vi "Traverse Cluster.vi"(10 "Nest Chain":string[](array[string]), 11 "Data Type":variant) -> (3 "Array":T1[](array[typedef]))   [LabVIEW 2023]
doc: "Reentrant VI recursively returns references of controls in a cluster and compiles data needed for display in tree, such as the nesting heirarchy of nested clusters."
uses:
  Cluster Element Description.ctl
  <vilib>/Utility/Data Type/NI_Data Type.lvlib
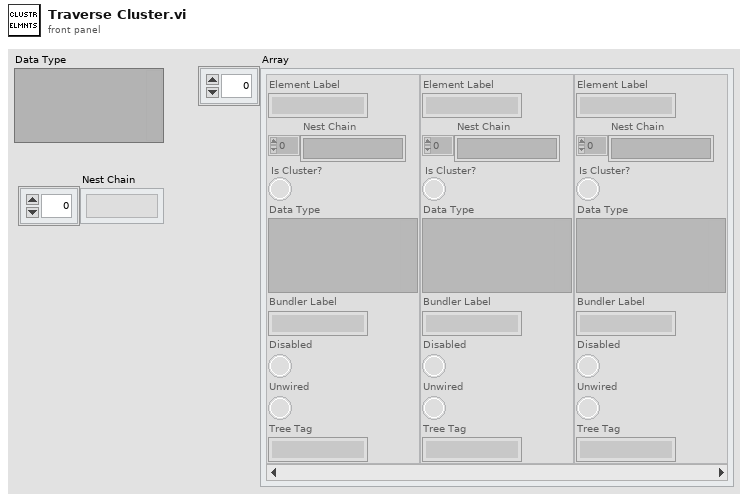
[diagram p1: front panel]
types:
  T1 = typedef "Cluster Element Description.ctl" = cluster{"Element Label":string, "Nest Chain":string[], "Is Cluster?":bool, "Data Type":variant, "Bundler Label":string, "Disabled":bool, "Unwired":bool, "Tree Tag":string}
  T2 = enum8{"Invalid Type", "Void", "I8", "I16", "I32", "I64", "U8", "U16", "U32", "U64", "Single Float", "Double Float", "Extended Float", "Single Complex", "Double Complex", "Extended Complex", "Enum U8", "Enum U16", "Enum U32", "Enum U64", "Single Float With Unit", "Double Float With Unit", "Extended Float With Unit", "Single Complex with Unit", "Double Complex with Unit", "Extended Complex with Unit", "Boolean", "String", "Path", "Picture", "Tag", "Array", "Cluster", "Variant", "LV Variant", "Waveform", "Timestamp", "Digital Waveform", "Digital Data", "ExpressData", "Refnum", "External Data", "VI", "Poly VI", "LabVIEW Class Instance", "Fixed Point"}
  T3 = typedef "NI_Data Type.lvlib/Data Type.ctl" = enum8{"Invalid Type", "Void", "I8", "I16", "I32", "I64", "U8", "U16", "U32", "U64", "Single Float", "Double Float", "Extended Float", "Single Complex", "Double Complex", "Extended Complex", "Enum U8", "Enum U16", "Enum U32", "Enum U64", "Single Float With Unit", "Double Float With Unit", "Extended Float With Unit", "Single Complex with Unit", "Double Complex with Unit", "Extended Complex with Unit", "Boolean", "String", "Path", "Picture", "Tag", "Array", "Cluster", "Variant", "LV Variant", "Waveform", "Timestamp", "Digital Waveform", "Digital Data", "ExpressData", "Refnum", "External Data", "VI", "Poly VI", "LabVIEW Class Instance", "Fixed Point", "Set Collection", "Map Collection"}
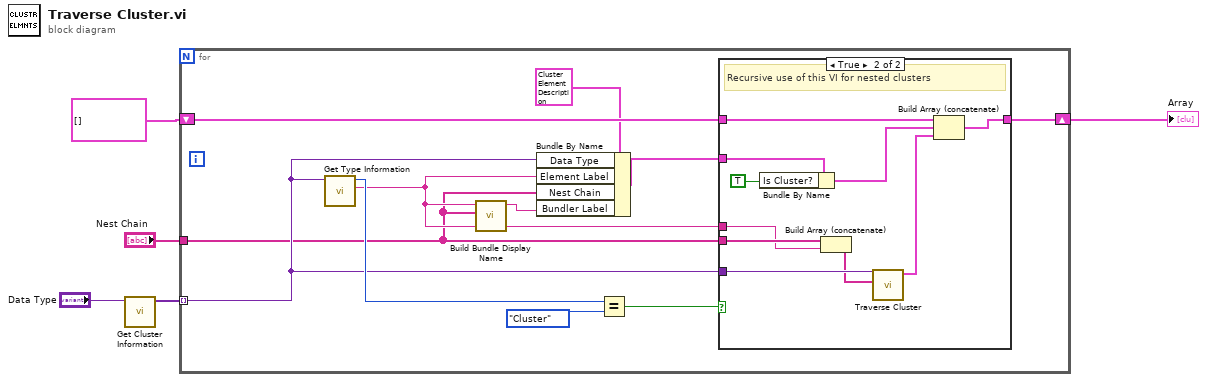
[diagram p0: block diagram]
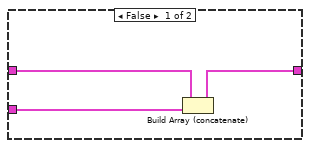
[diagram p2: hidden frame]
diagram:
  n1 = call <vilib>:"Get Cluster Information.vi"("variant"="Data Type") -> ("cluster elements"=w4:variant[])  [unwired: 9 in, 1 out]
  n2 = for {
    shift-right: [w11] -> w1
    shift-left: T1[] [] -> [w15]
    tunnel: w4 -> [w12] mode=indexing
    tunnel: "Nest Chain" -> [w9]
    n3 = call <vilib>:"Get Type Information.vi"("variant"=w12) -> ("name"=w10:string, "type"=w14:T3)  [unwired: 6 in, 3 out]
    n4 = call "Build Bundle Display Name.vi"("Nest Chain"=w9, "Element Label"=w10) -> ("Bundle display name"=w8:string)  [unwired: 9 in]
    n5 = Bundle By Name(cluster=T1 {"Element Label"="", "Nest Chain"=[], "Is Cluster?"=FALSE, "Data Type"=variant, "Bundler Label"="", "Disabled"=FALSE, "Unwired"=FALSE, "Tree Tag"=""} ("Cluster Element Data"), "Data Type"=w12, "Element Label"=w10, "Nest Chain"=w9, "Bundler Label"=w8) -> (w6:T1)
    n6 = Equal?(x=w14, y=T2."Cluster" ("type")) -> (x = y?=w16:bool)
    n7 = case shown="True" w16 {
      tunnel: [w18 w22] -> w11
      tunnel: w6 -> [w17 w28]
      tunnel: w15 -> [w19 w29]
      tunnel: w12 -> [_ w25]
      tunnel: w9 -> [_ w26]
      tunnel: w10 -> [_ w24]
      frame False {
        n8 = Build Array (concatenate)(w19, w17) -> (w18:T1[])
      }
      frame True {
        # "Recursive use of this VI for nested clusters"
        n9 = Bundle By Name(cluster=w28, "Is Cluster?"=TRUE) -> (w20:T1)
        n10 = Build Array (concatenate)(w26, w24) -> (w23:string[])
        n11 = call "Traverse Cluster.vi"("Nest Chain"=w23, "Data Type"=w25) -> ("Array"=w21:T1[])  [unwired: 9 in]
        n12 = Build Array (concatenate)(w29, w20, w21) -> (w22:T1[])
      }
    }
  }
  "Array" <- w1
